vi "Auto Main.vi"() -> ()   [LabVIEW 2020]
doc: "This template is for the Queued Message Handler design pattern.\n\nThe Event Handling Loop generates messages based on user interface actions.\n\nThe Message Handling Loop processes messages generated by the Event Handling Loop, or by other messages. The messages are string values, so new messages can be added easily to the Message Cases case structure in the Message Handling Loop. Each message cluster can also provide an optional value for Message Data, which is a variant that can be converted to whatever message-specific data is required."
uses:
  controls/Auto UI Data.ctl
  controls/Configuration Details.ctl
  <vilib>/vision/Image Controls.llb/IMAQ Image.ctl
  Database/Controls/DB Options.ctl
  IPC/MQTT/Controls/Publish data.ctl
  IPC/MQTT/Q Driver/Controls/IPC-MQTT-Q driver-Q Options.ctl
  support/Message Queue/Enqueue Message (Single).vi
  support/Message Queue/Auto Message Queue.lvlib
  support/User Event - Stop/Auto User Event - Stop.lvlib
panel:
  out "Shift Time":string
  out "User":string
  out "date/time string":string
  out "Shift":string
  in  "Multicolumn Listbox":i32(listbox)=-1
  out "Image Display":T1(plugin-control)
  out "Result":string
  out "Scanned Code":string
  out "Cycle Time (TAKT)":u16 caption="S"
  out "Variant":string
  out "Model":string
  out "TOTAL":dbl
  out "FAIL":dbl
  out "PASS":dbl
  in  "Error Status":string
  in  "Exit":bool
  in  "Actual Status":string
  out "Reset Seq":string
  # "AUTO RUN"
  # "Production Data"
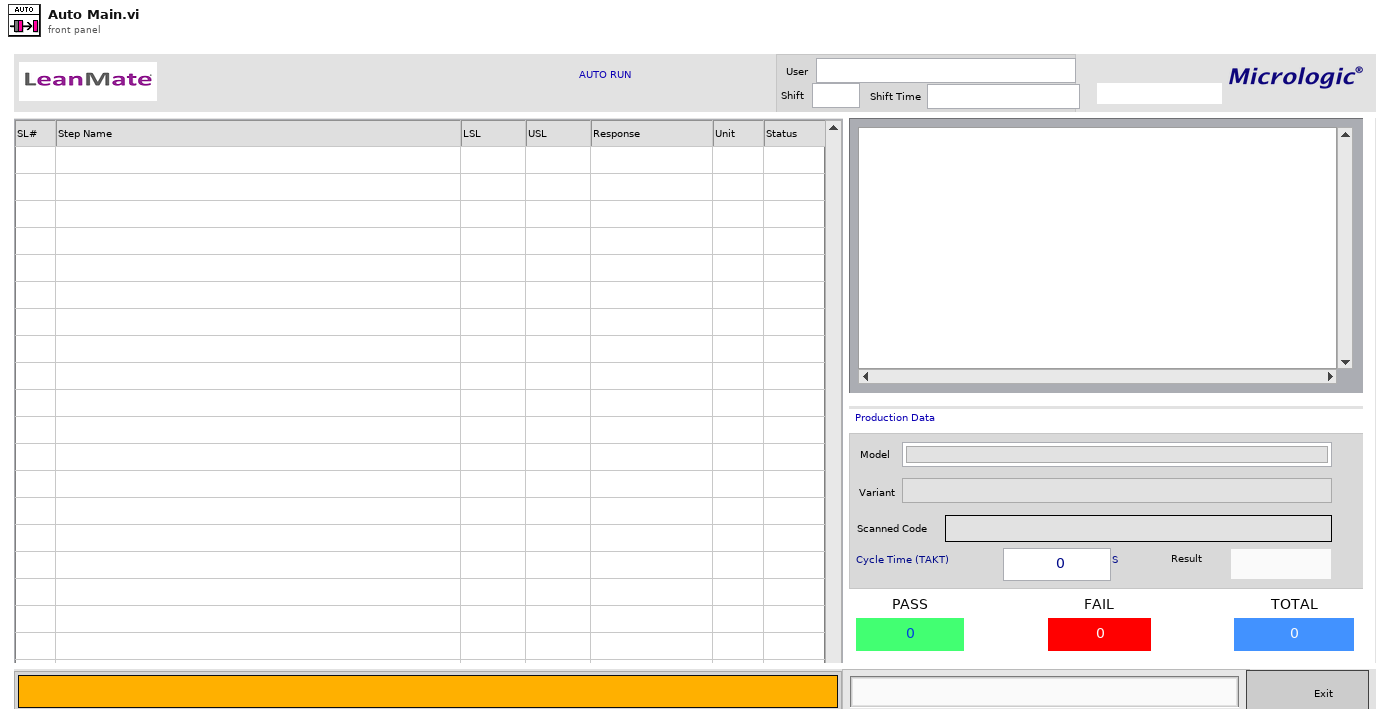
[diagram p1: front panel]
types:
  T1 = typedef "IMAQ Image.ctl" = refnum<image>
  T2 = enum32{"Invalid", "Standard", "Closed", "Hidden", "Minimized", "Maximized"}
  T3 = typedef "Auto UI Data.ctl" = cluster{"Status Mes":string, "Reset Status Ref":refnum<vi>, "Exit Button Ref":refnum<vi>, "Test List":refnum<vi>, "Actual Status":refnum<vi>, "Configuration":T4, "Model Name":string, "Variant Name":string, "Model Id":string, "Variant ID":string, "Error Status":refnum<vi>, "PASS COUNT":refnum<vi>, "FAIL COUNT":refnum<vi>, "TOTAL COUNT":refnum<vi>, "Result":refnum<vi>, "IO Names":cluster{"DI":string[], "DO":string[], "AI":string[], "AO":string[]}, "Image":T1, "Shift Info":string[][], "Start Time":timestamp, "Aborted?":bool, "Log Report":bool, "Report path":path, "Barcode":string, "Current Shift":string, "Station Name":string, "Actual Index":i32[], "Cycle Time?":bool, "exe":path, "Cycle Time (TAKT)":u16, "Test list index":u32, "Test index":u32[], "Part no":string}
  T4 = typedef "Configuration Details.ctl" = cluster{"SEQ_Config":cluster{"SEQ_Name":string, "Actual_SEQ":string[][], "Reset_SEQ":string[][]}[], "HW_Config":string[][], "DAQ_Config":string[][], "Salfty_Check_Inputs":string[][], "PLC_Config":string[][], "DAQ_Driver":string}
  T5 = typedef "Auto Message Queue.lvlib/All Message Queues.ctl" = cluster{"UI":refnum<queue>}
  T6 = typedef "DB Options.ctl" = enum16{"Select", "Execute", "Special Q", "Insert", "Update", "Delete", "Open", "Close"}
  T7 = enum32{"invalid app kind", "Development System", "Run Time System", "Student Edition", "Embedded LabVIEW", "Evaluation", "Custom"}
  T8 = typedef "Publish data.ctl" = cluster{"Topic":string, "Message":string}
  T9 = typedef "IPC-MQTT-Q driver-Q Options.ctl" = enum16{"En Q", "En Q N", "De Q", "Init", "En Q N Stack", "Flush", "Close"}
  T10 = typedef "Image Type" = u32
  T11 = typedef "Get Path - All Path Control.ctl" = cluster{"Source Code":path, "Exe":path, "data":path, "Dynamic VI's":path, "Plugable Drivers":path, "Error Logs":path, "Database":path, "Squence":path}
  T12 = cluster{"SEQ_Name":string, "Actual_SEQ":string[][], "Reset_SEQ":string[][]}[]
  T13 = cluster{"SEQ_Name":string, "Actual_SEQ":string[][], "Reset_SEQ":string[][]}
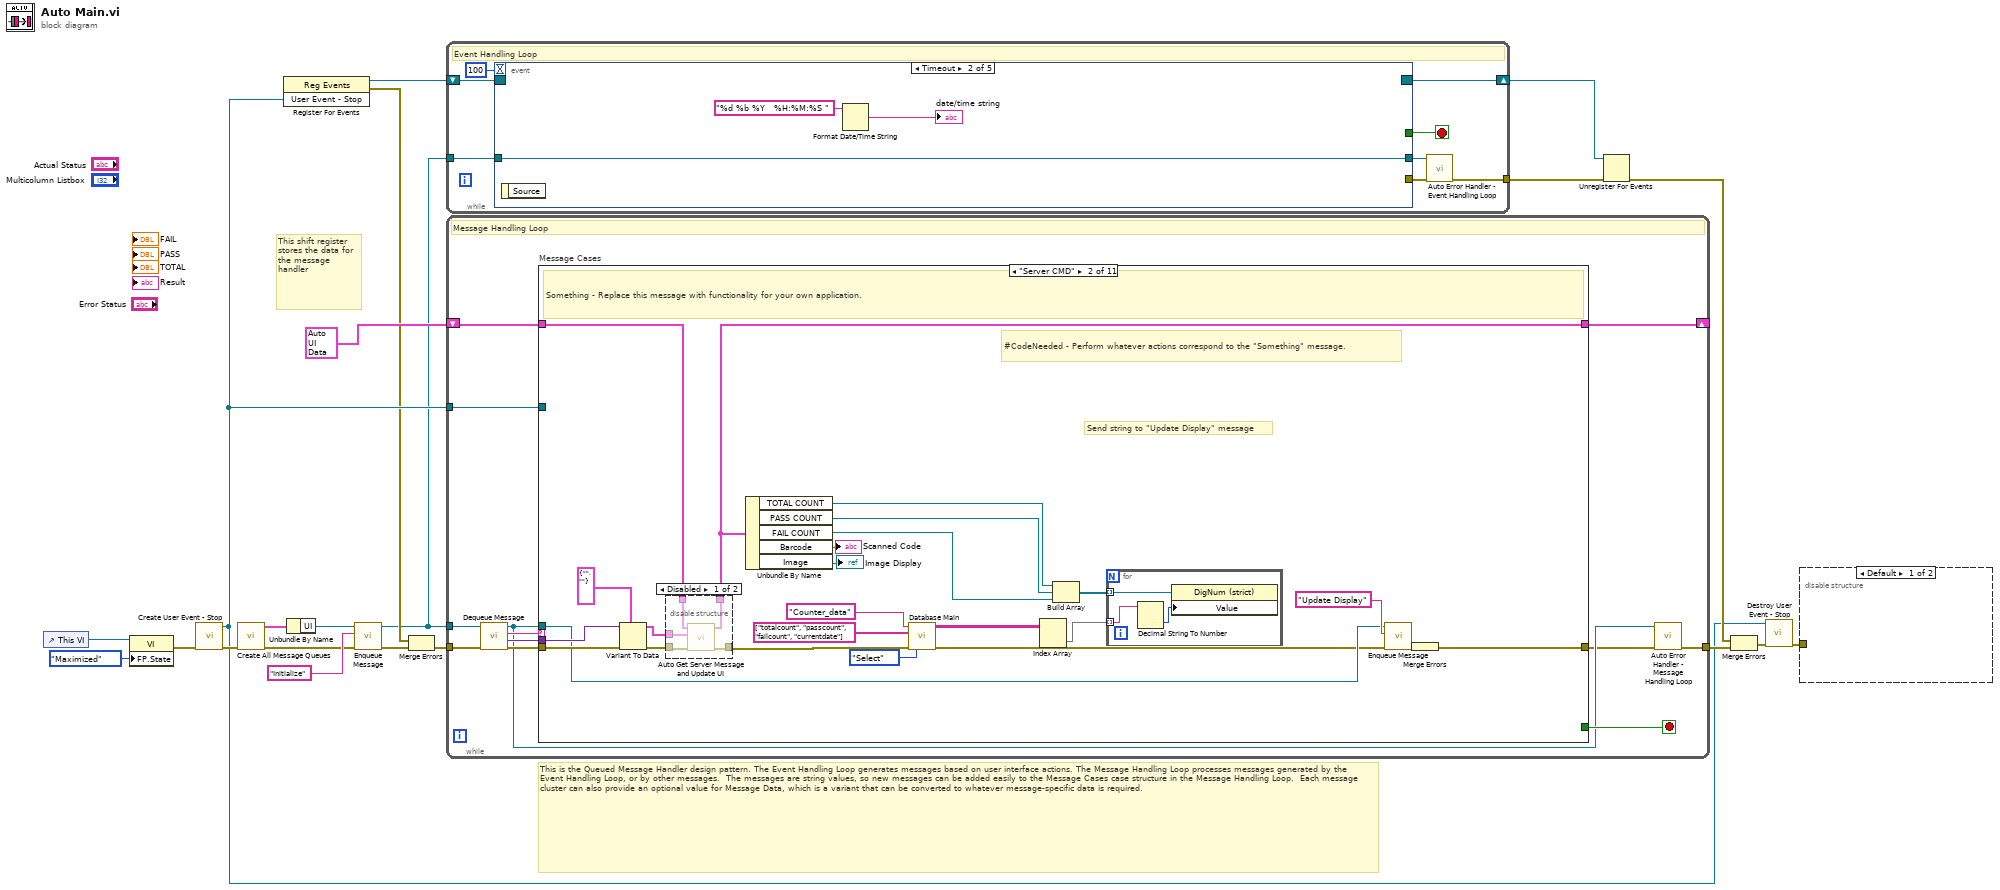
[diagram p0: block diagram]
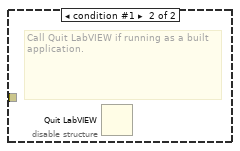
[diagram p2: hidden frame]
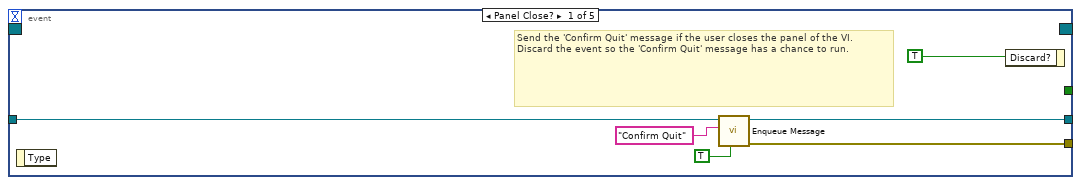
[diagram p3: hidden frame]
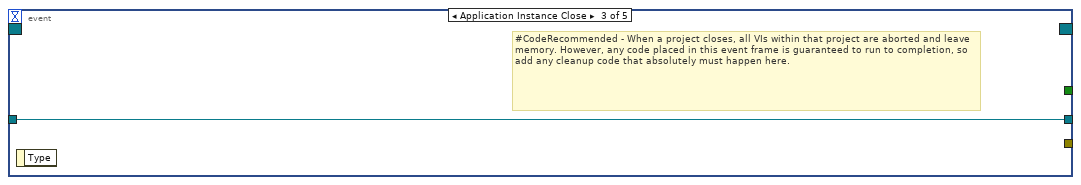
[diagram p4: hidden frame]
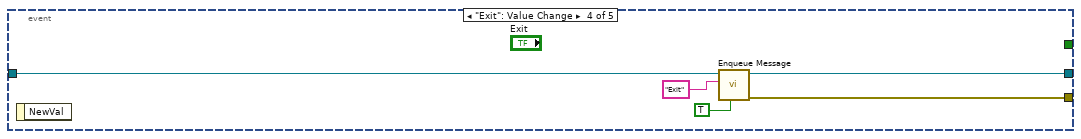
[diagram p5: hidden frame]
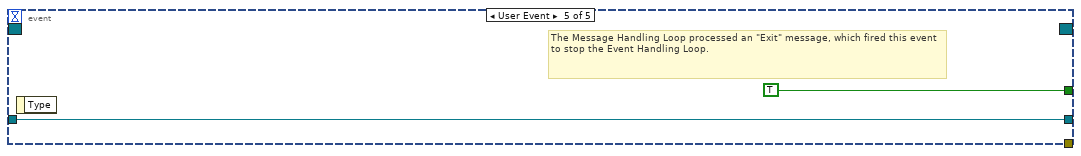
[diagram p6: hidden frame]
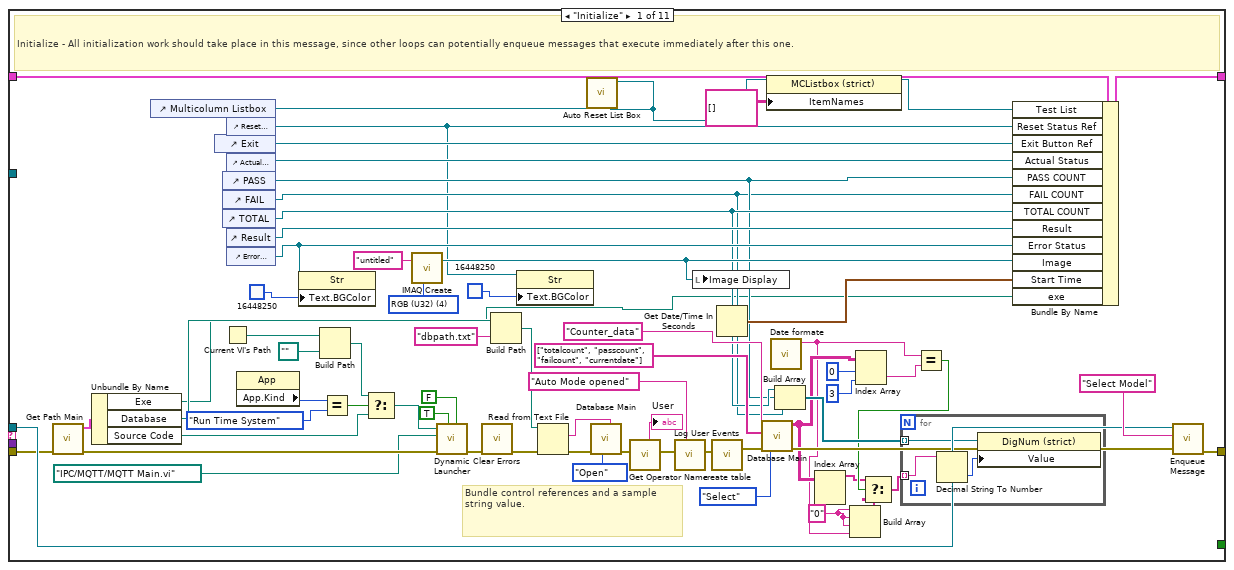
[diagram p7: hidden frame]
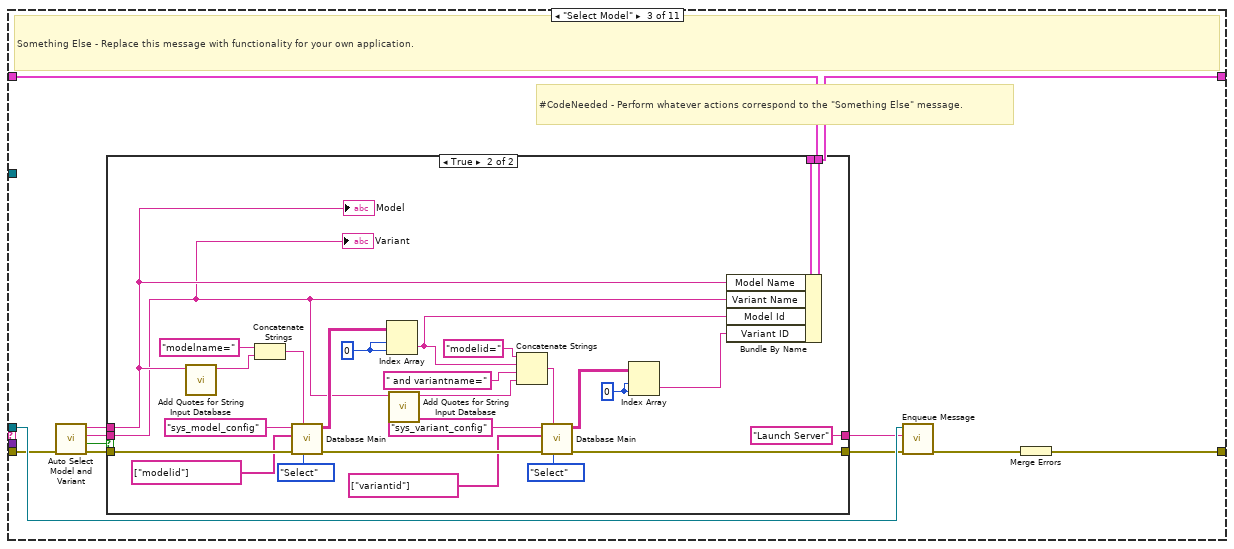
[diagram p9: hidden frame]
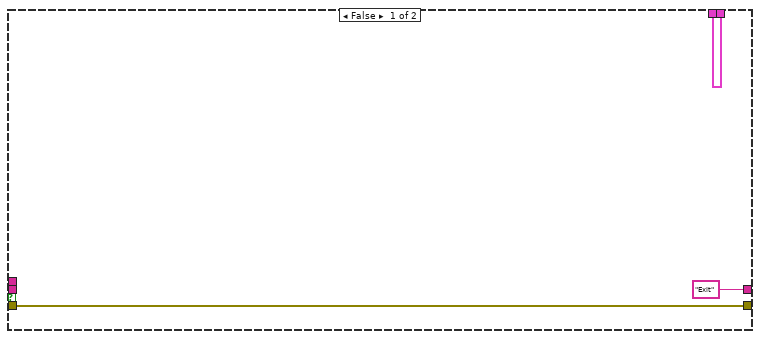
[diagram p10: hidden frame]
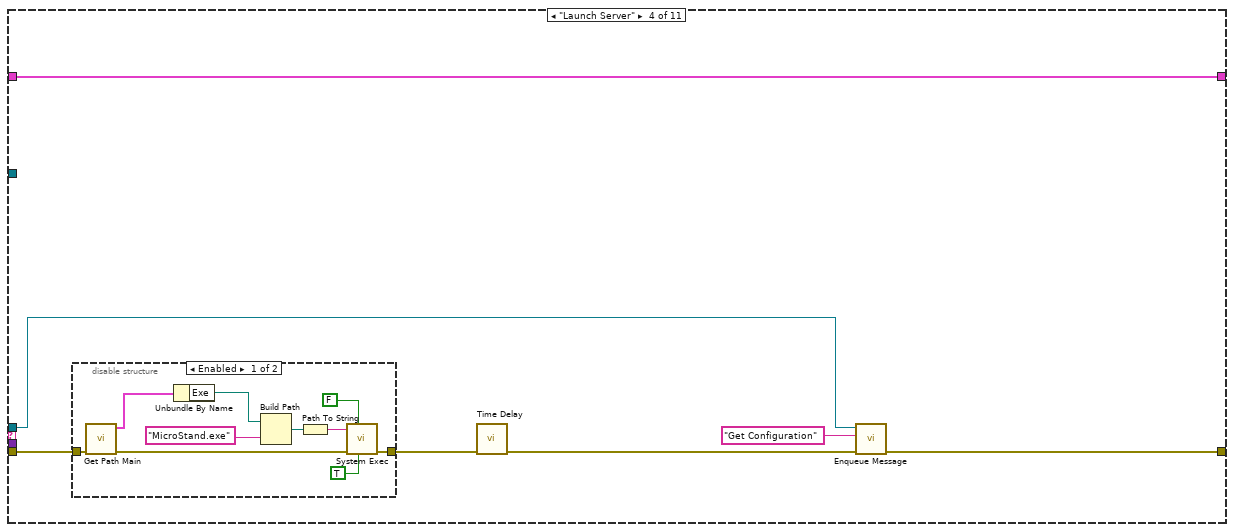
[diagram p11: hidden frame]
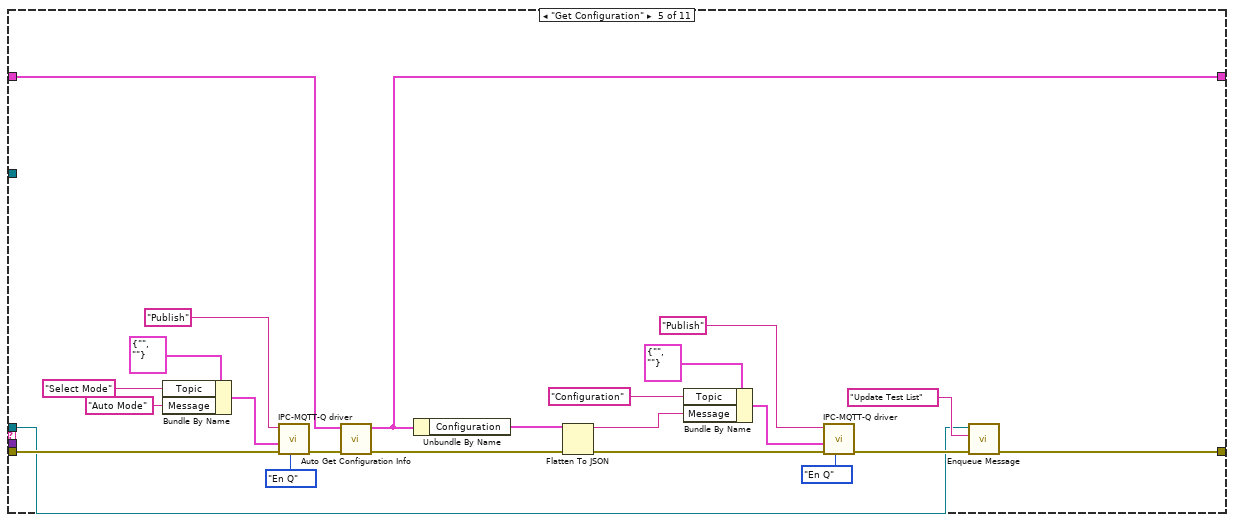
[diagram p13: hidden frame]
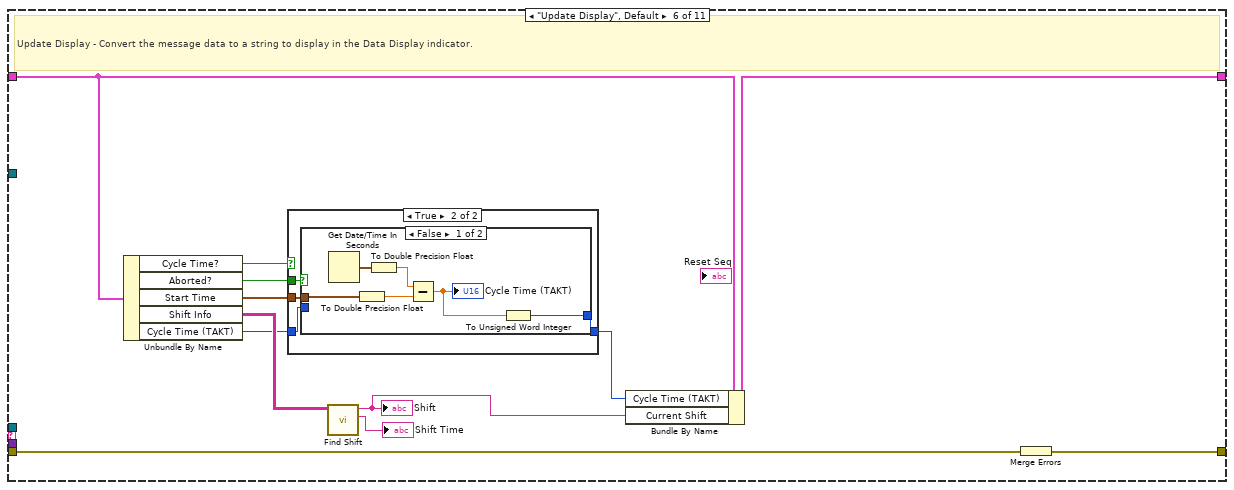
[diagram p14: hidden frame]
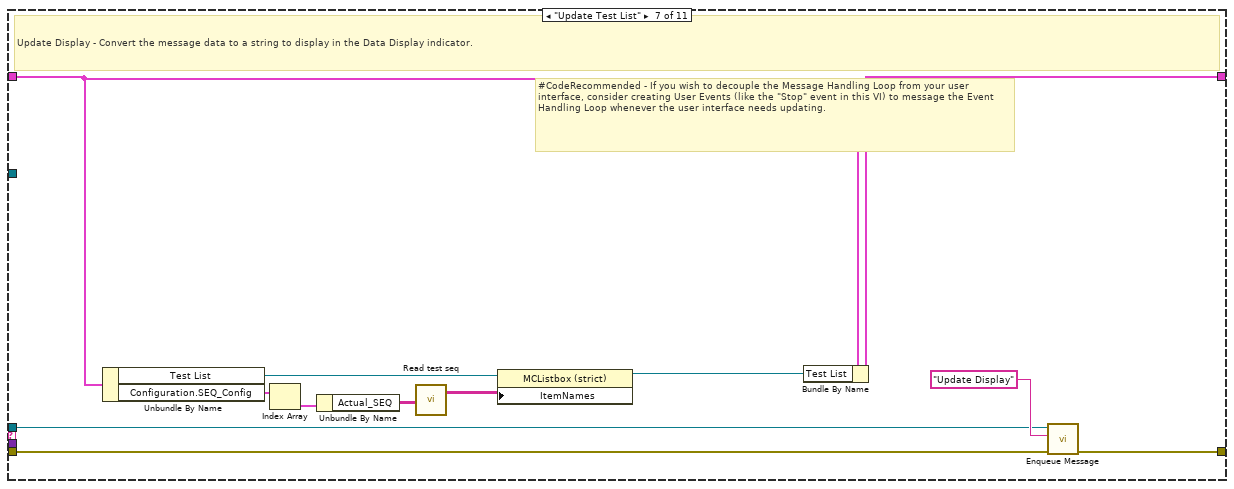
[diagram p17: hidden frame]
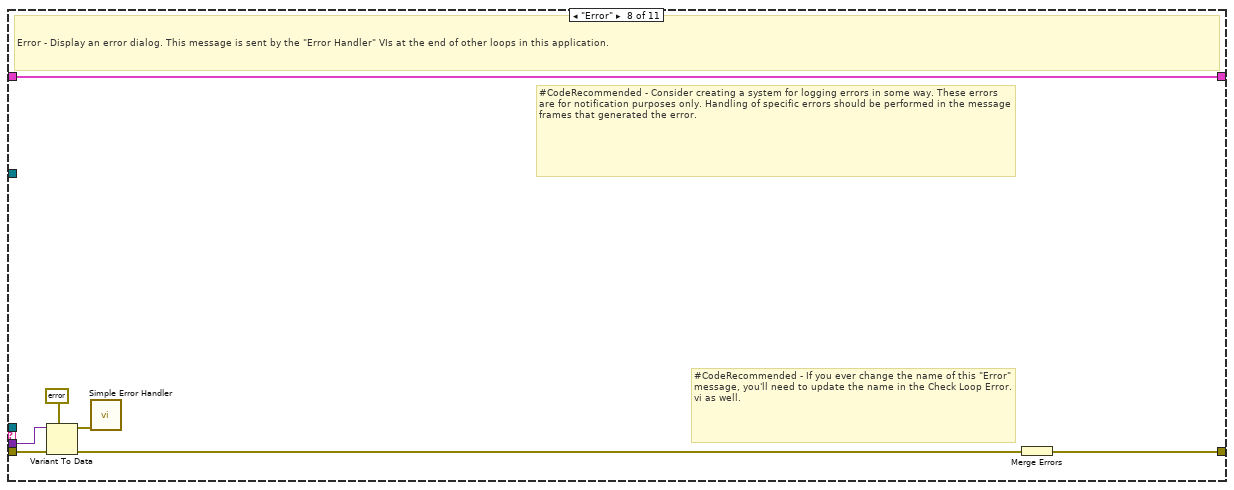
[diagram p18: hidden frame]
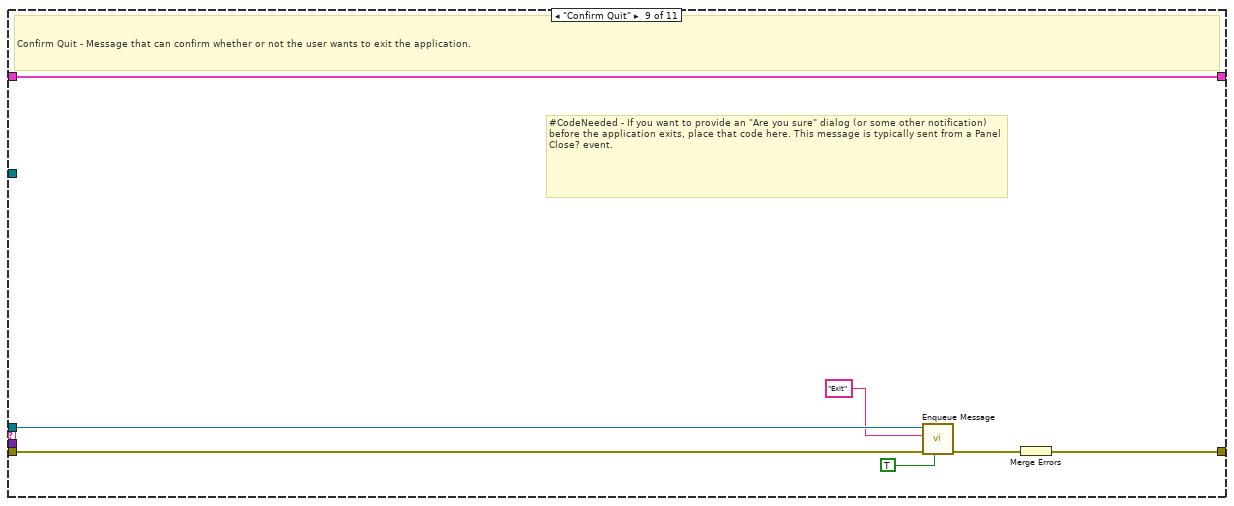
[diagram p19: hidden frame]
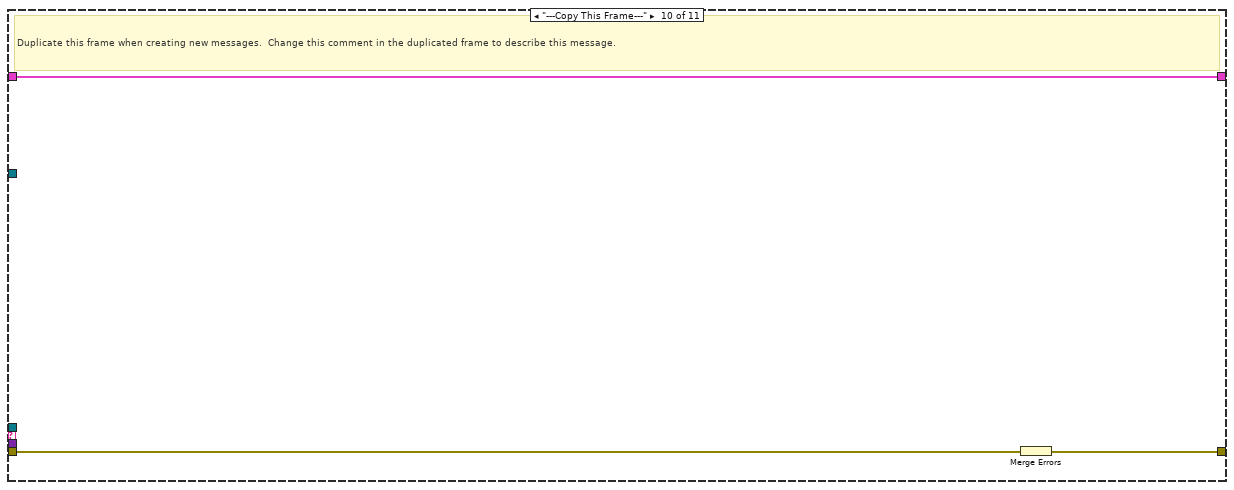
[diagram p20: hidden frame]
diagram:
  # "This is the Queued Message Handler design pattern. The Event Handling Loop generates messages based on user interface actions. The Message Handling Loop processes messages generated by the Event Handling Loop, or by other messages.  The messages are string values, so new messages can be added easily to the Message Cases case structure in the Message Handling Loop.  Each message cluster can also provide an optional value for Message Data, which is a variant that can be converted to whatever message-specific data is required."
  # "This shift register stores the data for the message handler"
  n1 = control-ref of="This VI"() -> (w3:refnum<vi>)
  n2 = property class="VI"(reference=w3, "FP.State"=T2."Maximized" ("Front Panel Window:State")) -> (error out=w1:errorcluster)  [unwired: 1 in, 1 out]
  n3 = call "Create User Event - Stop.vi"("error in (no error)"=w1) -> ("error out"=w19:errorcluster, "User Event - Stop"=w11:refnum<user-event>)  [unwired: 9 in]
  n4 = call "Create All Message Queues.vi"("error in (no error)"=w19) -> ("error out"=w5:errorcluster, "Message Queues out"=w21:T5)  [unwired: 9 in]
  n5 = register-events(w11) -> (reference out=w12:refnum<event-registration>, error out=w9:errorcluster)  [unwired: 2 in]
  n6 = Unbundle By Name(w21) -> ("UI"=w7:refnum<queue>)
  n7 = call-poly "Enqueue Message.vi"("error in (no error)"=w5, "Message"="Initialize", "Message Queue"=w7) -> ("error out"=w4:errorcluster, "dup Message Queue"=w6:refnum<queue>)  [unwired: 7 in]
  n8 = Merge Errors(w9, w4) -> (w10:errorcluster)
  n9 = while {
    tunnel: w6 -> [w25]
    shift-right: [w32] -> _
    shift-left: T3 {"Status Mes"="", "Reset Status Ref"=refnum, "Exit Button Ref"=refnum, "Test List"=refnum, "Actual Status"=refnum, "Configuration"={"SEQ_Config"=[], "HW_Config"=[], "DAQ_Config"=[], "Salfty_Check_Inputs"=[], "PLC_Config"=[], "DAQ_Driver"=""}, "Model Name"="", "Variant Name"="", "Model Id"="", "Variant ID"="", "Error Status"=refnum, "PASS COUNT"=refnum, "FAIL COUNT"=refnum, "TOTAL COUNT"=refnum, "Result"=refnum, "IO Names"={"DI"=[], "DO"=[], "AI"=[], "AO"=[]}, "Image"=refnum, "Shift Info"=[], "Start Time"=timestamp(0 s since 1904-01-01), "Aborted?"=FALSE, "Log Report"=FALSE, "Report path"=path "", "Barcode"="", "Current Shift"="", "Station Name"="", "Actual Index"=[], "Cycle Time?"=FALSE, "exe"=path "", "Cycle Time (TAKT)"=0, "Test list index"=0, "Test index"=[], "Part no"=""} ("Data Cluster") -> [w33]
    tunnel: w11 -> [w30]
    tunnel: w10 -> [w29]
    tunnel: [w23] -> w20
    stop <- w31 stop-if-true
    # "Message Handling Loop"
    n10 = call "Dequeue Message.vi"("error in (no error)"=w29, "Message Queue"=w25) -> ("error out"=w28:errorcluster, "Message Data"=w26:variant, "Message"=w27:string, "dup Message Queue"=w24:refnum<queue>)  [unwired: 6 in]
    n11 = case "Message Cases" shown="\"Server CMD\"" w27 {
      tunnel: w24 -> [w94 w115 w144 w180 w194 _ w243 _ w262 _ w295]
      tunnel: w28 -> [w93 w125 w143 w182 w201 w220 w242 w259 w266 w269 w290]
      tunnel: [w99 w126 w146 w181 w195 w228 w241 w253 w264 w267 w293] -> w22
      tunnel: w33 -> [w98 w119 w136 w183 w216 w227 w252 w258 w265 w268 w270]
      tunnel: [w97 w118 w135 w183 w214 w222 w251 w258 w265 w268 w270] -> w32
      tunnel: [_ _ _ _ _ _ _ _ _ _ TRUE] -> w31
      tunnel: w26 -> [_ w123 _ _ _ _ _ w257 _ _ w287]
      tunnel: w30 -> [_ _ _ _ _ _ _ _ _ _ w292]
      frame "Initialize" {
        w40 = "0"
        w71 = T10 4 items=["Grayscale (U8)", "Grayscale (I16)", "Grayscale (SGL)", "Complex (CSG)", "RGB (U32)", "HSL (U32)", "RGB (U64)", "Grayscale (U16)"] ("Image Type")
        # "Bundle control references and a sample string value."
        # "Initialize - All initialization work should take place in this message, since other loops can potentially enqueue messages that execute immediately after this one."
        n12 = call "Get Path Main.vi"("error in (no error)"=w93) -> ("error out"=w91:errorcluster, "All Path"=w92:T11)  [unwired: 9 in]
        n13 = Unbundle By Name(w92) -> ("Exe"=w49:path, "Database"=w67:path, "Source Code"=w76:path)
        n14 = control-ref of="Multicolumn Listbox"() -> (w36:refnum<vi>)
        n15 = control-ref of="Exit"() -> (w96:refnum<vi>)
        n16 = control-ref of="PASS"() -> (w51:refnum<vi>)
        n17 = control-ref of="FAIL"() -> (w50:refnum<vi>)
        n18 = control-ref of="TOTAL"() -> (w52:refnum<vi>)
        n19 = Current VI's Path() -> (path=w75:path)
        n20 = control-ref of="Reset Status"() -> (w37:refnum<vi>)
        n21 = control-ref of="Actual Status"() -> (w87:refnum<vi>)
        n22 = control-ref of="Result"() -> (w82:refnum<vi>)
        n23 = control-ref of="Error Status"() -> (w60:refnum<vi>)
        n24 = property class="App"() -> ("App.Kind"=w81:T7)  [unwired: 2 in, 2 out]
        n25 = property class="Str"(reference=w60, "Text.BGColor"=u32 16448250) -> ()  [unwired: 1 in, 2 out]
        n26 = Build Path(base path=w75, name or relative path=path ".." ("path")) -> (appended path=w77:path)
        n27 = Equal?(x=w81, y=T7."Run Time System") -> (x = y?=w78:bool)
        n28 = Select(t=w77, s=w78, f=w76) -> (s? t:f=w68:path)
        n29 = call "IMAQ Create"("Image Name"="untitled", "Image Type"=w71) -> ("New Image"=w70:T1)  [unwired: 3 in, 1 out]
        n30 = call "Dynamic Launcher.vi"("Wait Until Done"=FALSE, "Auto Dispose Reference"=TRUE, "error in (no error)"=w91, "Dynamic VI's"=path "IPC/MQTT/MQTT Main.vi", "Folder path"=w68) -> ("error out"=w73:errorcluster)  [unwired: 5 in, 1 out]
        n31 = call <vilib>:"Clear Errors.vi"("error in (no error)"=w73) -> ("error out"=w69:errorcluster)  [unwired: 5 in, 1 out]
        n32 = Build Path(base path=w67, name or relative path="dbpath.txt") -> (appended path=w74:path)
        n33 = property class="Str"(reference=w37, "Text.BGColor"=u32 16448250) -> ()  [unwired: 1 in, 2 out]
        n34 = Read from Text File(file (use dialog)=w74, error in=w69) -> (text=w84:string, error out=w86:errorcluster)  [unwired: 2 in, 2 out]
        n35 = call "Auto Reset List Box.vi"("MulticolumnListbox in"=w36) -> ()  [unwired: 10 in, 1 out]
        n36 = call "Database Main.vi"("DB Name/Path"=w84, "Option"=DB_Options."Open", "error in (no error)"=w86) -> ("error out"=w65:errorcluster)  [unwired: 6 in, 2 out]
        n37 = call "Get Operator Name.vi"("error in (no error)"=w65) -> ("error out"=w64:errorcluster, "Operator Name"=→"User":string)  [unwired: 9 in]
        n38 = call "Log User Events.vi"("Log Message"="Auto Mode opened", "error in (no error)"=w64) -> ("error out"=w61:errorcluster)  [unwired: 9 in]
        n39 = local write "Image Display"(w70) -> ()
        n40 = call "create table.vi"("error in"=w61) -> ("error out"=w55:errorcluster)  [unwired: 10 in]
        n41 = Get Date/Time In Seconds() -> (seconds since 1Jan1904=w66:timestamp)
        n42 = call "Database Main.vi"("Option"=DB_Options."Select", "error in (no error)"=w55, "Column Name"=string[] ["totalcount", "passcount", "failcount", "currentdate"], "table Name/Query"="Counter_data") -> ("error out"=w54:errorcluster, "Data"=w45:string[][])  [unwired: 5 in, 1 out]
        n43 = property class="MCListbox (strict)"(reference=w36, "ItemNames"=string[][] [] ("Item Names")) -> (reference out=w34:refnum<vi>)  [unwired: 1 in, 1 out]
        n44 = call "Date formate.vi"() -> ("date string 2"=w41:string)  [unwired: 11 in]
        n45 = Build Array(w52, w51, w50) -> (w53:refnum<vi>[])
        n46 = Index Array(array=w45) -> (element=w43:string[])  [unwired: 2 in]
        n47 = Build Array(w40, w40, w40, w41) -> (w39:string[])
        n48 = Index Array(array=w45, index (row)=0 ("disabled index (row)"), index (col)=3 ("disabled index (col)")) -> (element=w48:string)
        n49 = Equal?(x=w41, y=w48) -> (x = y?=w44:bool)
        n50 = Select(t=w43, s=w44, f=w39) -> (s? t:f=w42:string[])
        n51 = for {
          tunnel: w53 -> [w102] mode=indexing
          tunnel: w42 -> [w101] mode=indexing
          n52 = Decimal String To Number(string=w101) -> (number=w100:i32)  [unwired: 2 in, 1 out]
          n53 = property class="DigNum (strict)"(reference=w102, "Value"=w100) -> ()  [unwired: 1 in, 2 out]
        }
        n54 = Bundle By Name(cluster=w98, "Test List"=w34, "Reset Status Ref"=w37, "Exit Button Ref"=w96, "Actual Status"=w87, "PASS COUNT"=w51, "FAIL COUNT"=w50, "TOTAL COUNT"=w52, "Result"=w82, "Error Status"=w60, "Image"=w70, "Start Time"=w66, "exe"=w49) -> (w97:T3)
        n55 = call-poly "Enqueue Message.vi"("error in (no error)"=w54, "Message"="Select Model", "Message Queue"=w94) -> ("error out"=w99:errorcluster)  [unwired: 7 in, 1 out]
      }
      frame "Server CMD" {
        # "Send string to \"Update Display\" message"
        # "#CodeNeeded - Perform whatever actions correspond to the \"Something\" message."
        # "Something - Replace this message with functionality for your own application."
        n56 = Variant To Data(error in=w125, type=T8 {"Topic"="", "Message"=""} ("Cluster"), Variant=w123) -> (data=w122:T8, error out=w121:errorcluster)
        n57 = disable-structure shown="Disabled" {
          disable-tunnel: w122 -> [w131 _]
          disable-tunnel: w121 -> [w130 _]
          disable-tunnel: w119 -> [w129 _]
          disable-tunnel: [w128 _] -> w118
          disable-tunnel: [w127 _] -> w106
          frame Disabled {
            n58 = call "Auto Get Server Message and Update UI.vi"("error in (no error)"=w130, "MQTT Data"=w131, "Data Cluster"=w129) -> ("error out"=w127:errorcluster, "Data Out"=w128:T3)  [unwired: 7 in]
          }
          frame Enabled {
          }
        }
        n59 = Unbundle By Name(w118) -> ("TOTAL COUNT"=w110:refnum<vi>, "PASS COUNT"=w109:refnum<vi>, "FAIL COUNT"=w108:refnum<vi>, "Barcode"=→"Scanned Code":string, "Image"=→"Image Display":T1)
        n60 = call "Database Main.vi"("Option"=DB_Options."Select", "error in (no error)"=w106, "Column Name"=string[] ["totalcount", "passcount", "failcount", "currentdate"], "table Name/Query"="Counter_data") -> ("error out"=w105:errorcluster, "Data"=w104:string[][])  [unwired: 5 in, 1 out]
        n61 = Index Array(array=w104) -> (element=w103:string[])  [unwired: 2 in]
        n62 = Build Array(w110, w109, w108) -> (w107:refnum<vi>[])
        n63 = for {
          tunnel: w107 -> [w134] mode=indexing
          tunnel: w103 -> [w133] mode=indexing
          n64 = Decimal String To Number(string=w133) -> (number=w132:i32)  [unwired: 2 in, 1 out]
          n65 = property class="DigNum (strict)"(reference=w134, "Value"=w132) -> ()  [unwired: 1 in, 2 out]
        }
        n66 = call-poly "Enqueue Message.vi"("error in (no error)"=w105, "Message"="Update Display", "Message Queue"=w115) -> ("error out"=w116:errorcluster)  [unwired: 7 in, 1 out]
        n67 = Merge Errors(w116) -> (w126:errorcluster)
      }
      frame "Select Model" {
        # "#CodeNeeded - Perform whatever actions correspond to the \"Something Else\" message."
        # "Something Else - Replace this message with functionality for your own application."
        n68 = call "Auto Select Model and Variant.vi"("error in (no error)"=w143) -> ("error out"=w138:errorcluster, "Ok"=w142:bool, "Vaiant Selected"=w139:string, "Model Selected"=w141:string)  [unwired: 7 in]
        n69 = case shown="True" w142 {
          tunnel: ["Exit" ("f") "Launch Server" ("f")] -> w140
          tunnel: w141 -> [_ w151]
          tunnel: w139 -> [_ w150]
          tunnel: w138 -> [w147 w174]
          tunnel: [w147 w162] -> w137
          tunnel: w136 -> [w148 w176]
          tunnel: [w148 w175] -> w135
          frame False {
          }
          frame True {
            w155 = 0 ("index (row)")
            w166 = 0 ("index (row)")
            n70 = call "Add Quotes for String Input Database.vi"("String in"=w151) -> ("String Out"=w168:string)  [unwired: 10 in]
            n71 = Concatenate Strings("modelname=" ("Where"), w168) -> (w169:string)
            n72 = call "Database Main.vi"("Option"=DB_Options."Select", "Where"=w169, "error in (no error)"=w174, "Column Name"=string[] ["modelid"], "table Name/Query"="sys_model_config") -> ("error out"=w163:errorcluster, "Data"=w167:string[][])  [unwired: 4 in, 1 out]
            n73 = Index Array(array=w167, index (row)=w166, index (col)=w166) -> (element=w158:string)
            n74 = call "Add Quotes for String Input Database.vi"("String in"=w150) -> ("String Out"=w156:string)  [unwired: 10 in]
            n75 = Concatenate Strings("modelid=" ("Where"), w158, " and variantname=" ("string"), w156) -> (w159:string)
            n76 = call "Database Main.vi"("Option"=DB_Options."Select", "Where"=w159, "error in (no error)"=w163, "Column Name"=string[] ["variantid"], "table Name/Query"="sys_variant_config") -> ("error out"=w162:errorcluster, "Data"=w154:string[][])  [unwired: 4 in, 1 out]
            n77 = Index Array(array=w154, index (row)=w155, index (col)=w155) -> (element=w153:string)
            n78 = Bundle By Name(cluster=w176, "Model Name"=w151, "Variant Name"=w150, "Model Id"=w158, "Variant ID"=w153) -> (w175:T3)
            "Model" <- w151
            "Variant" <- w150
          }
        }
        n79 = call-poly "Enqueue Message.vi"("error in (no error)"=w137, "Message"=w140, "Message Queue"=w144) -> ("error out"=w145:errorcluster)  [unwired: 7 in, 1 out]
        n80 = Merge Errors(w145) -> (w146:errorcluster)
      }
      frame "Launch Server" {
        n81 = disable-structure shown="Enabled" {
          disable-tunnel: w182 -> [w193 _]
          disable-tunnel: [w184 _] -> w178
          frame Enabled {
            n82 = call "Get Path Main.vi"("error in (no error)"=w193) -> ("error out"=w190:errorcluster, "All Path"=w189:T11)  [unwired: 9 in]
            n83 = Unbundle By Name(w189) -> ("Exe"=w188:path)
            n84 = Build Path(base path=w188, name or relative path="MicroStand.exe") -> (appended path=w186:path)
            n85 = Path To String(path=w186) -> (string=w185:string)
            n86 = call <vilib>:"System Exec.vi"("run minimized? (F)"=TRUE, "wait until completion? (T)"=FALSE, "error in (no error)"=w190, "command line"=w185) -> ("error out"=w184:errorcluster)  [unwired: 4 in, 3 out]
          }
          frame Disabled {
          }
        }
        n87 = call "Time Delay"("error in (no error)"=w178) -> ("error out"=w177:errorcluster)  [unwired: 10 in]
        n88 = call-poly "Enqueue Message.vi"("error in (no error)"=w177, "Message"="Get Configuration", "Message Queue"=w180) -> ("error out"=w181:errorcluster)  [unwired: 7 in, 1 out]
      }
      frame "Get Configuration" {
        n89 = Bundle By Name(cluster=T8 {"Topic"="", "Message"=""} ("Cluster"), "Topic"="Select Mode", "Message"="Auto Mode") -> (w210:T8)
        n90 = call "IPC-MQTT-Q driver.vi"("Q Options"=IPC-MQTT-Q_driver-Q_Options."En Q", "error in (no error)"=w201, "Message Data"=w210, "Message"="Publish") -> ("error out"=w200:errorcluster)  [unwired: 5 in, 2 out]
        n91 = call "Auto Get Configuration Info.vi"("error in (no error)"=w200, "Data Cluster in"=w216) -> ("error out"=w215:errorcluster, "Data Cluster out"=w214:T3)  [unwired: 8 in]
        n92 = Unbundle By Name(w214) -> ("Configuration"=w213:T4)
        n93 = Flatten To JSON(anything=w213, error in (no error)=w215) -> (JSON string=w198:string, 11:w199:errorcluster)  [unwired: 1 in]
        n94 = Bundle By Name(cluster=T8 {"Topic"="", "Message"=""} ("Cluster"), "Topic"="Configuration", "Message"=w198) -> (w206:T8)
        n95 = call "IPC-MQTT-Q driver.vi"("Q Options"=IPC-MQTT-Q_driver-Q_Options."En Q", "error in (no error)"=w199, "Message Data"=w206, "Message"="Publish") -> ("error out"=w196:errorcluster)  [unwired: 5 in, 2 out]
        n96 = call-poly "Enqueue Message.vi"("error in (no error)"=w196, "Message"="Update Test List", "Message Queue"=w194) -> ("error out"=w195:errorcluster)  [unwired: 7 in, 1 out]
      }
      frame "Update Display", Default {
        # "Update Display - Convert the message data to a string to display in the Data Display indicator."
        n97 = Unbundle By Name(w227) -> ("Cycle Time?"=w219:bool, "Aborted?"=w225:bool, "Start Time"=w224:timestamp, "Shift Info"=w226:string[][], "Cycle Time (TAKT)"=w217:u16)
        n98 = case shown="True" w219 {
          tunnel: w225 -> [_ w233]
          tunnel: w224 -> [_ w232]
          tunnel: [w229 w231] -> w218
          tunnel: w217 -> [w229 w230]
          frame False {
          }
          frame True {
            n99 = case shown="False" w233 {
              tunnel: w232 -> [w239 _]
              tunnel: [w234 w240] -> w231
              tunnel: w230 -> [_ w240]
              frame False {
                n100 = Get Date/Time In Seconds() -> (seconds since 1Jan1904=w238:timestamp)
                n101 = To Double Precision Float(number=w239) -> (double precision float=w236:dbl)
                n102 = To Double Precision Float(number=w238) -> (double precision float=w237:dbl)
                n103 = Subtract(x=w237, y=w236) -> (x-y=w235:dbl)
                "Cycle Time (TAKT)" <- w235
                n104 = To Unsigned Word Integer(number=w235) -> (unsigned 16bit integer=w234:u16)
              }
              frame True {
              }
            }
          }
        }
        n105 = call "Find Shift.vi"("Shift Info"=w226) -> ("Shift Time"=→"Shift Time":string, "Shift Name"=w221:string)  [unwired: 9 in]
        "Shift" <- w221
        n106 = Bundle By Name(cluster=w227, "Cycle Time (TAKT)"=w218, "Current Shift"=w221) -> (w222:T3)
        n107 = Merge Errors(w220) -> (w228:errorcluster)
      }
      frame "Update Test List" {
        # "#CodeRecommended - If you wish to decouple the Message Handling Loop from your user interface, consider creating User Events (like the \"Stop\" event in this VI) to message the Event Handling Loop whenever the user interface needs updating."
        # "Update Display - Convert the message data to a string to display in the Data Display indicator."
        n108 = Unbundle By Name(w252) -> ("Test List"=w247:refnum<vi>, "Configuration.SEQ_Config"=w250:T12)
        n109 = Index Array(array=w250) -> (element=w249:T13)  [unwired: 1 in]
        n110 = Unbundle By Name(w249) -> ("Actual_SEQ"=w248:string[][])
        n111 = call "Read test seq.vi"("In data"=w248) -> ("Out Data"=w246:string[][])  [unwired: 2 in]
        n112 = property class="MCListbox (strict)"(reference=w247, "ItemNames"=w246) -> (reference out=w245:refnum<vi>)  [unwired: 1 in, 1 out]
        n113 = Bundle By Name(cluster=w252, "Test List"=w245) -> (w251:T3)
        n114 = call-poly "Enqueue Message.vi"("error in (no error)"=w242, "Message"="Update Display", "Message Queue"=w243) -> ("error out"=w241:errorcluster)  [unwired: 7 in, 1 out]
      }
      frame "Error" {
        # "#CodeRecommended - If you ever change the name of this \"Error\" message, you'll need to update the name in the Check Loop Error.vi as well."
        # "#CodeRecommended - Consider creating a system for logging errors in some way. These errors are for notification purposes only. Handling of specific errors should be performed in the message frames that generated the error."
        # "Error - Display an error dialog. This message is sent by the \"Error Handler\" VIs at the end of other loops in this application."
        n115 = Variant To Data(error in=w259, type=errorcluster {"status"=FALSE, "code"=0, "source"=""} ("error constant"), Variant=w257) -> (data=w255:errorcluster, error out=w254:errorcluster)
        n116 = call <vilib>:"Simple Error Handler.vi"("error in (no error)"=w255) -> ()  [unwired: 4 in, 5 out]
        n117 = Merge Errors(w254) -> (w253:errorcluster)
      }
      frame "Confirm Quit" {
        # "#CodeNeeded - If you want to provide an \"Are you sure\" dialog (or some other notification) before the application exits, place that code here. This message is typically sent from a Panel Close? event."
        # "Confirm Quit - Message that can confirm whether or not the user wants to exit the application."
        n118 = call-poly "Enqueue Message.vi"("Priority Message? (F)"=TRUE, "error in (no error)"=w266, "Message"="Exit", "Message Queue"=w262) -> ("error out"=w263:errorcluster)  [unwired: 6 in, 1 out]
        n119 = Merge Errors(w263) -> (w264:errorcluster)
      }
      frame "---Copy This Frame---" {
        # "Duplicate this frame when creating new messages.  Change this comment in the duplicated frame to describe this message."
        n120 = Merge Errors(w269) -> (w267:errorcluster)
      }
      frame "Exit" {
        # "Stop the VI"
        # "Release the message queue reference"
        # "#CodeNeeded - Add any required cleanup code here. Note that if 'Exit' was called as a result of an error, an error dialog will be displayed. Add any custom error handling for an 'Exit' condition here as well."
        # "Exit - Exit the application."
        n121 = Variant To Data(type=errorcluster {"status"=FALSE, "code"=0, "source"=""} ("error constant"), Variant=w287) -> (data=w288:errorcluster)  [unwired: 1 in, 1 out]
        n122 = call <vilib>:"Simple Error Handler.vi"("error in (no error)"=w288) -> ()  [unwired: 4 in, 5 out]
        n123 = Release Queue(queue=w295, error in (no error)=w290) -> (error out=w271:errorcluster)  [unwired: 1 in, 2 out]
        n124 = Bundle By Name(cluster=T8 {"Topic"="", "Message"=""} ("Cluster"), "Topic"="Client CMD", "Message"="Exit") -> (w275:T8)
        n125 = call "Database Main.vi"("Option"=DB_Options."Close", "error in (no error)"=w271) -> ("error out"=w281:errorcluster)  [unwired: 7 in, 2 out]
        n126 = call "IPC-MQTT-Q driver.vi"("Q Options"=IPC-MQTT-Q_driver-Q_Options."En Q", "error in (no error)"=w281, "Message Data"=w275, "Message"="Publish") -> ("error out"=w280:errorcluster)  [unwired: 5 in, 2 out]
        n127 = call "IPC-MQTT-Q driver.vi"("Q Options"=IPC-MQTT-Q_driver-Q_Options."En Q", "error in (no error)"=w280, "Message Data"="Exit" ("Message"), "Message"="cmd") -> ("error out"=w274:errorcluster)  [unwired: 5 in, 2 out]
        n128 = call "Fire User Event - Stop.vi"("User Event - Stop"=w292) -> ("error out"=w291:errorcluster)  [unwired: 10 in]
        n129 = call "Log User Events.vi"("Log Message"="Auto Mode closed", "error in (no error)"=w274) -> ("error out"=w273:errorcluster)  [unwired: 9 in]
        n130 = Merge Errors(w291, w273) -> (w293:errorcluster)
      }
    }
    n131 = call "Auto Error Handler - Message Handling Loop.vi"("error in (no error)"=w22, "Message Queue"=w24) -> ("dup error in"=w23:errorcluster)  [unwired: 8 in, 1 out]
  }
  n132 = while {
    tunnel: w6 -> [w303]
    shift-right: [w301] -> w16
    shift-left: w12 -> [w302]
    tunnel: [w297] -> w13
    stop <- w299 stop-if-true
    # "Event Handling Loop"
    n133 = event shown="[1] Timeout" {
      selector: w302 -> [_ _ _ _ _]
      dyn-events: [_ _ _ _ _] -> w301
      timeout: 100 -> [_ _ _ _ _]
      tunnel: [_ _ _ _ TRUE ("Discard?")] -> w299
      tunnel: w303 -> [w308 w312 w313 w318 w320]
      tunnel: [w307 _ _ w317 _] -> w300
      tunnel: [w306 w312 w313 w316 w320] -> w298
      event Panel Close? {
        # "Send the 'Confirm Quit' message if the user closes the panel of the VI. Discard the event so the 'Confirm Quit' message has a chance to run."
        n134 = event-data() -> ()  [unwired: 1 in, 1 out]
        n135 = call-poly "Enqueue Message.vi"("Priority Message? (F)"=TRUE, "Message"="Confirm Quit", "Message Queue"=w308) -> ("error out"=w307:errorcluster, "dup Message Queue"=w306:refnum<queue>)  [unwired: 7 in]
        n136 = event-data("Discard?"=TRUE) -> ()  [unwired: 1 in, 1 out]
      }
      event Timeout {
        n137 = event-data() -> ()  [unwired: 1 in, 1 out]
        n138 = Format Date/Time String(time format string (%c)="%d %b %Y   %H:%M:%S ") -> (date/time string=→"date/time string":string)  [unwired: 2 in]
      }
      event Application Instance Close {
        # "#CodeRecommended - When a project closes, all VIs within that project are aborted and leave memory. However, any code placed in this event frame is guaranteed to run to completion, so add any cleanup code that absolutely must happen here."
        n139 = event-data() -> ()  [unwired: 1 in, 1 out]
      }
      event "Exit": Value Change {
        n140 = event-data() -> ()  [unwired: 1 in, 1 out]
        n141 = call-poly "Enqueue Message.vi"("Priority Message? (F)"=TRUE, "Message"="Exit", "Message Queue"=w318) -> ("error out"=w317:errorcluster, "dup Message Queue"=w316:refnum<queue>)  [unwired: 7 in]
      }
      event User Event {
        # "The Message Handling Loop processed an \"Exit\" message, which fired this event to stop the Event Handling Loop."
        n142 = event-data() -> ()  [unwired: 1 in, 1 out]
      }
    }
    n143 = call "Auto Error Handler - Event Handling Loop.vi"("error in (no error)"=w300, "Message Queue"=w298) -> ("dup error in"=w297:errorcluster)  [unwired: 8 in, 1 out]
  }
  n144 = Unregister For Events(event registration refnum=w16, error in=w13) -> (error out=w17:errorcluster)
  n145 = Merge Errors(w17, w20) -> (w18:errorcluster)
  n146 = call "Destroy User Event - Stop.vi"("error in (no error)"=w18, "User Event - Stop"=w11) -> ("error out"=w14:errorcluster)  [unwired: 9 in]
  n147 = disable-structure shown="Default" {
    disable-tunnel: w14 -> [_ _]
    frame condition #0 (active) {
    }
    frame condition #1 {
      # "Call Quit LabVIEW if running as a built application."
      n148 = Quit LabVIEW() -> ()  [unwired: 1 in]
    }
  }
